vi "Tof3v5.vi"() -> ()   [LabVIEW 2013]
uses:
  <vilib>/Analysis/baseanly.llb/Mean (DBL).vi
  <vilib>/Analysis/NI_AAL_SigProc.lvlib
  <vilib>/ptbypt/NI_PtbyPt.lvlib
  <vilib>/Analysis/NI_AALBase.lvlib
panel:
  out "velocities":dbl(graph)
  out "peak 2 start":dbl
  out "peak 1 start":dbl
  in  "Filename":path=path "test.lvm"
  in  "Enable":bool=TRUE
  out "data":dynamicdata(graph)
  in  "stop":bool
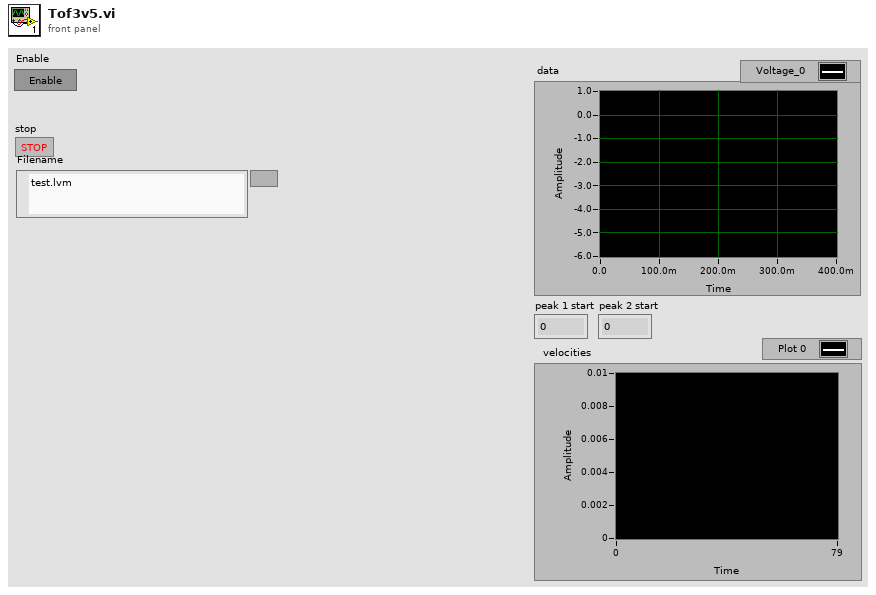
[diagram p1: front panel]
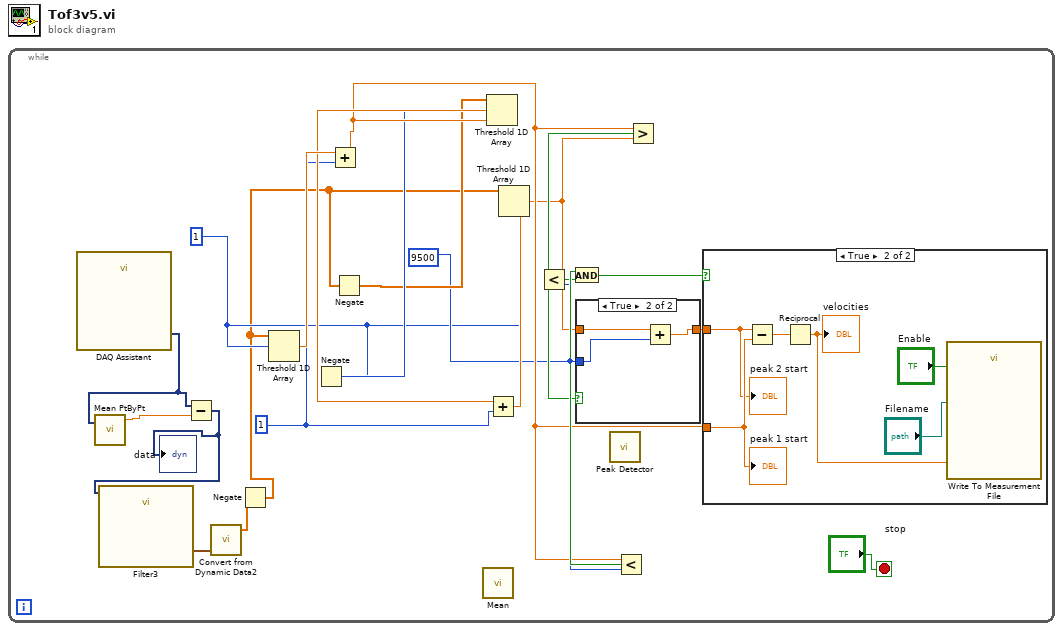
[diagram p0: block diagram]
diagram:
  n1 = while {
    stop <- "stop" stop-if-true
    w11 = 1
    w8 = 9500
    w7 = 1
    n2 = call "DAQ Assistant"() -> ("data"=w4:dynamicdata)  [unwired: 17 in, 2 out]
    n3 = call <vilib>:"Mean PtByPt.vi"("x"=w4) -> ("mean"=w5:dbl)  [unwired: 3 in, 1 out]
    n4 = Subtract(x=w4, y=w5) -> (x-y=w1:dynamicdata)
    "data" <- w1
    n5 = call "Filter3"("input signal"=w1) -> ("filtered data"=w6:waveform(dbl))  [unwired: 17 in, 1 out]
    n6 = call "Convert from Dynamic Data2"("Dynamic Data Type"=w6) -> ("Array"=w3:dbl[])  [unwired: 3 in]
    n7 = Negate(x=w3) -> (-x=w2:dbl[])
    n8 = Threshold 1D Array(2:w7, 3:w2) -> (0:w18:dbl)  [unwired: 1 in]
    n9 = Negate(x=w7) -> (-x=w10:i32)
    n10 = Add(x=w18, y=w11) -> (x+y=w15:dbl)
    n11 = Negate(x=w2) -> (-x=w9:dbl[])
    n12 = call-poly <vilib>:"Mean.vi"() -> ()  [unwired: 1 in, 2 out]
    n13 = Threshold 1D Array(1:w15, 2:w10, 3:w9) -> (0:w17:dbl)
    n14 = Add(x=w17, y=w11) -> (x+y=w16:dbl)
    n15 = Threshold 1D Array(1:w16, 2:w7, 3:w2) -> (0:w13:dbl)
    n16 = Less?(x=w13, y=w8) -> (x < y?=w20:bool)
    n17 = call <vilib>:"Peak Detector.vi"() -> ()  [unwired: 7 in, 5 out]
    n18 = Less?(x=w15, y=w8) -> (x < y?=w21:bool)
    n19 = And(x=w21, y=w20) -> (x .and. y?=w19:bool)
    n20 = Greater?(x=w15, y=w13) -> (0:w14:bool)
    n21 = case shown="True" w14 {
      tunnel: w13 -> [w23 w26]
      tunnel: [w23 w25] -> w12
      tunnel: w8 -> [_ w24]
      frame False {
      }
      frame True {
        n22 = Add(x=w26, y=w24) -> (x+y=w25:dbl)
      }
    }
    n23 = case shown="True" w19 {
      tunnel: w15 -> [_ w32]
      tunnel: w12 -> [_ w31]
      frame False {
      }
      frame True {
        n24 = Subtract(x=w31, y=w32) -> (x-y=w30:dbl)
        n25 = Reciprocal(x=w30) -> (1/x=w27:dbl)
        "velocities" <- w27
        n26 = call "Write To Measurement File"("Signals"=w27, "Enable"="Enable", "Filename"="Filename") -> ()  [unwired: 14 in, 3 out]
        "peak 1 start" <- w32
        "peak 2 start" <- w31
      }
    }
  }
